vi "Execute.vi"(8 "error in (no error)":errorcluster, 10 "Abstract Consumer in":refnum<class "Abstract Consumer.lvclass">, 11 "Log Word Message in":refnum<class "Log Message.lvclass">) -> (0 "error out":errorcluster, 1 "Abstract Response out":refnum<class "Abstract Response Message.lvclass">, 2 "Abstract Consumer out":refnum<class "Abstract Consumer.lvclass">, 3 "Log Word Message out":refnum<class "Log Message.lvclass">, 4 "Stop?":bool)   [LabVIEW 2020, in "AIM ARINC 429 Engine.lvlib" / "Implementation.lvlib" / "Word Logging.lvlib" / "Log Message.lvclass"]
uses:
  Log Message.lvclass
  <vilib>/NI/VeriStand Custom Device Messaging/Consumer/Abstract Consumer/Abstract Consumer.lvclass
  <vilib>/NI/VeriStand Custom Device Messaging/Message/Abstract Response Message/Abstract Response Message.lvclass
  Logger Interface/Logger Interface.lvclass
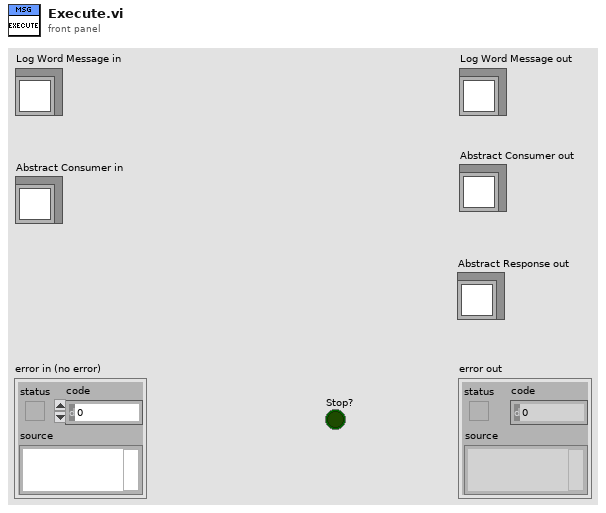
[diagram p1: front panel]
types:
  T1 = typedef "AIM ARINC 429 Engine.lvlib/Implementation.lvlib/Word Logging.lvlib/Logger Data Reference.ctl" = refnum<data-value>
  T2 = typedef "Ballard ARINC 429 Engine.lvlib/Implementation.lvlib/Logging.lvlib/Word.ctl" = cluster{"message info":cluster{"hardware channel":u8, "label":u8, "SDI":u8}, "data word":u32, "time stamp":dbl}
  T3 = cluster{"Logger Interface":refnum<class "Logger Interface.lvclass">}
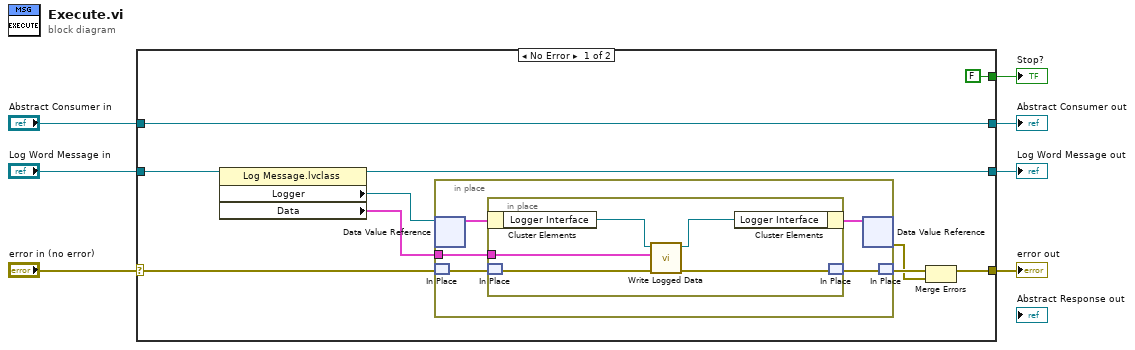
[diagram p0: block diagram]
diagram:
  n1 = case shown="No Error" "error in (no error)" {
    selector: "error in (no error)" -> [w12 w30]
    tunnel: [w9 w30] -> w6
    tunnel: [w17 w28] -> w5
    tunnel: "Abstract Consumer in" -> [w17 w28]
    tunnel: [FALSE ("Stop?") _] -> w3
    tunnel: [w13 w29] -> w2
    tunnel: "Log Word Message in" -> [w15 w29]
    frame No Error {
      n2 = property class="Log Message.lvclass"(reference=w15) -> (reference out=w13:refnum<class "Log Message.lvclass">, "Logger"=w10:T1, "Data"=w14:T2[])  [unwired: 1 in, 1 out]
      n3 = in-place {
        in-place-border: w14 -> [w22]
        n4 = in-place-dvr #1(w10) -> (w19:T3)  [unwired: 1 out]
        n5 = in-place-match #2(w12) -> (w21:errorcluster)
        n6 = in-place {
          in-place-border: w22 -> [w27]
          n7 = in-place-cluster #3(w19) -> ("Logger Interface"=w24:refnum<class "Logger Interface.lvclass">)
          n8 = in-place-match #4(w21) -> (w26:errorcluster)
          n9 = call-dynamic "Write Logged Data.vi"("error in (no error)"=w26, "Data"=w27, "Logger Interface in"=w24) -> ("error out"=w25:errorcluster, "Logger Interface out"=w23:refnum<class "Logger Interface.lvclass">)  [unwired: 7 in]
          n10 = in-place-cluster #3("Logger Interface"=w23) -> (w18:T3)
          n11 = in-place-match #4(w25) -> (w20:errorcluster)
        }
        n12 = in-place-dvr #1(w18) -> (w8:errorcluster)  [unwired: 1 out]
        n13 = in-place-match #2(w20) -> (w11:errorcluster)
      }
      n14 = Merge Errors(w11, w8) -> (w9:errorcluster)
    }
    frame Error {
    }
  }
  "error out" <- w6
  "Log Word Message out" <- w2
  "Abstract Consumer out" <- w5
  "Stop?" <- w3
